vi "commit VI reference.vi"(8 "error in":errorcluster, 10 "VI Refnum in":refnum<vi>, 11 "io configuration in":refnum<class "io configuration.lvclass">) -> (0 "error out":errorcluster, 2 "VI Refnum out":refnum<vi>, 3 "io configuration out":refnum<class "io configuration.lvclass">)   [LabVIEW 2015, in "io configuration.lvclass"]
doc: "Sets properties of the class using a VI reference."
uses:
  io configuration.lvclass
  io configuration.lvclass/io configuration.ctl
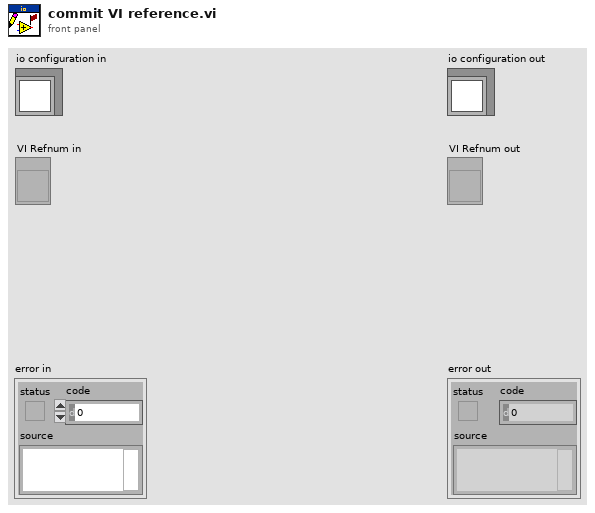
[diagram p1: front panel]
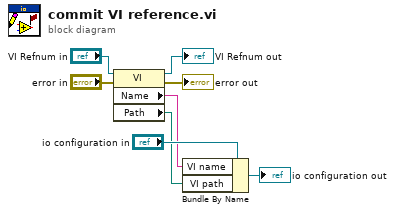
[diagram p0: block diagram]
diagram:
  n1 = property class="VI"(reference="VI Refnum in", error in="error in") -> (reference out=→"VI Refnum out":refnum<vi>, error out=→"error out":errorcluster, "Name"=w1:string, "Path"=w2:path)
  n2 = Bundle By Name(cluster="io configuration in", "VI name"=w1, "VI path"=w2) -> (→"io configuration out":refnum<class "io configuration.lvclass">)
